vi "Red Tail.vi"(8 "error in (no error)":errorcluster, 11 "CIPC Reference":u64) -> (0 "error out":errorcluster, 3 "Tail":u32)   [LabVIEW 2021, in "CIF_NI_CIPC.lvlib"]
uses:
  CIF_NI_CIPC.lvlib
  libnicipc.dll
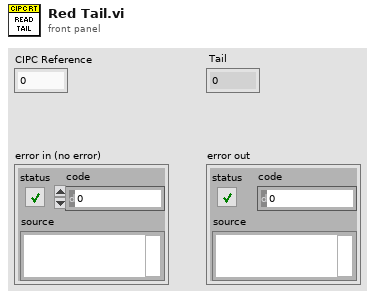
[diagram p1: front panel]
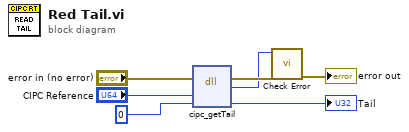
[diagram p0: block diagram]
diagram:
  n1 = dll-call lib="libnicipc.*" fn="cipc_getTail"(error in="error in (no error)", "cipc_buffer_ref"="CIPC Reference", "tail"=u32 0 ("head")) -> (error out=w6:errorcluster, "return type"=w5:i32, "tail"=→"Tail":u32)  [unwired: 3 in, 1 out]
  n2 = call "Check Error.vi"("error in (no error)"=w6, "Error Code"=w5) -> ("error out"=→"error out":errorcluster)  [unwired: 9 in]
